vi "SSC Digital Configure HRAM Settings.vi"(0 "Digital SSC in":T1[](array[typedef]), 1 "Number of Samples is Finite":bool=TRUE, 5 "Cycles to Acquire":i32(ring)=2303 items=["Failed Cycles"=2303, "All Cycles"=2304], 7 "Pretrigger Samples":i32, 9 "Buffer Size Per Site":i64=32000, 11 "error in":errorcluster, 12 "Max Samples To Acquire Per Site":i32=8191) -> (4 "Digital SSC out":T1[](array[typedef]), 15 "error out":errorcluster)   [LabVIEW 2020]
doc: "Uses the start label you specify to burst the pattern on the pin(s) and pin group(s) you specify."
uses:
  SSC Digital.ctl
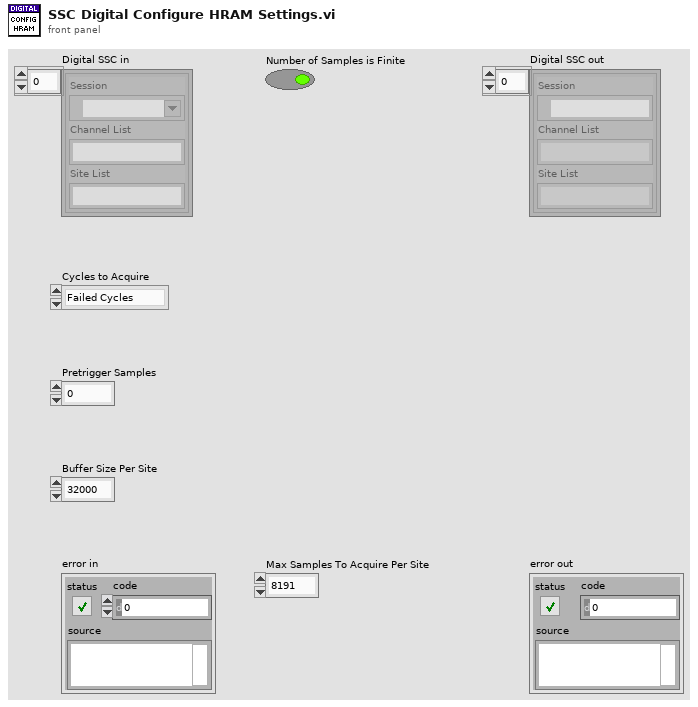
[diagram p1: front panel]
types:
  T1 = typedef "SSC Digital.ctl" = cluster{"Session":refnum<k15>, "Channel List":string, "Site List":string}
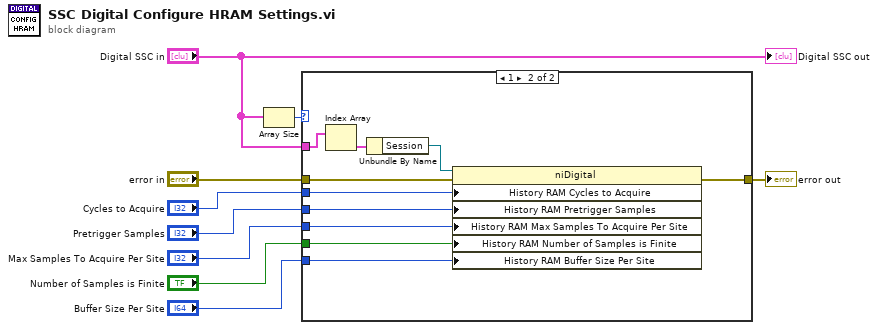
[diagram p0: block diagram]
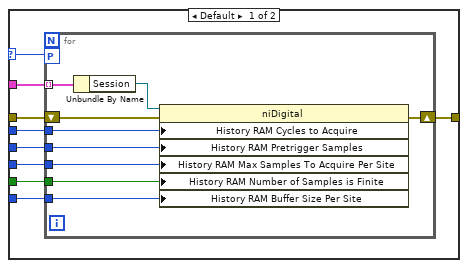
[diagram p2: hidden frame]
diagram:
  n1 = Array Size(array="Digital SSC in") -> (size(s)=w8:i32)
  n2 = case shown="1" w8 {
    selector: w8 -> [w18 _]
    tunnel: "error in" -> [w16 w36]
    tunnel: "Digital SSC in" -> [w17 w37]
    tunnel: "Cycles to Acquire" -> [w15 w35]
    tunnel: "Pretrigger Samples" -> [w14 w34]
    tunnel: "Max Samples To Acquire Per Site" -> [w13 w33]
    tunnel: "Number of Samples is Finite" -> [w12 w32]
    tunnel: "Buffer Size Per Site" -> [w11 w31]
    tunnel: [w10 w30] -> w1
    frame Default {
      n3 = for {
        tunnel: w17 -> [w27] mode=indexing
        workers-P: w18 -> [_]
        tunnel: w15 -> [w23]
        tunnel: w14 -> [w22]
        tunnel: w13 -> [w21]
        tunnel: w12 -> [w20]
        tunnel: w11 -> [w19]
        shift-right: [w26] -> w10
        shift-left: w16 -> [w24]
        n4 = Unbundle By Name(w27) -> ("Session"=w25:refnum<k15>)
        n5 = property class="niDigital"(reference=w25, error in=w24, "History RAM Cycles to Acquire"=w23, "History RAM Pretrigger Samples"=w22, "History RAM Max Samples To Acquire Per Site"=w21, "History RAM Number of Samples is Finite"=w20, "History RAM Buffer Size Per Site"=w19) -> (error out=w26:errorcluster)  [unwired: 1 out]
      }
    }
    frame 1 {
      n6 = Index Array(array=w37) -> (element=w28:T1)  [unwired: 1 in]
      n7 = Unbundle By Name(w28) -> ("Session"=w29:refnum<k15>)
      n8 = property class="niDigital"(reference=w29, error in=w36, "History RAM Cycles to Acquire"=w35, "History RAM Pretrigger Samples"=w34, "History RAM Max Samples To Acquire Per Site"=w33, "History RAM Number of Samples is Finite"=w32, "History RAM Buffer Size Per Site"=w31) -> (error out=w30:errorcluster)  [unwired: 1 out]
    }
  }
  "error out" <- w1
  "Digital SSC out" <- "Digital SSC in"
